vi "Graph_FPGA_v00.vi"() -> ()   [LabVIEW 2010]
doc: "Controls 6 phase locks based on the interference of two beams at a beam-splitter."
uses:
  Strict Type Defs/Graph Errors.ctl
  Strict Type Defs/Graph Lock Point.ctl
  Strict Type Defs/Graph Output.ctl
  Strict Type Defs/Control Graph Input.ctl
  Strict Type Defs/PII individual.ctl
  Strict Type Defs/Error Scale Graph.ctl
  Strict Type Defs/Lock Thresh Graph.ctl
  Strict Type Defs/Theta graph.ctl
  Strict Type Defs/Safety First.ctl
  Strict Type Defs/Scope.ctl
  Strict Type Defs/Graph Max.ctl
  Strict Type Defs/Graph Min.ctl
  <vilib>/eio/EIONode/EIONode.xnode
  <vilib>/rvi/eio/nirviEIOImplementation/nirviEIOImplementation.xnode
  <vilib>/rvi/eio/common/nirviEmuClasses.ctl
  <vilib>/rvi/DataTransferAndStorage/Container/XNode/niFpgaContainer.xnode
  <vilib>/rvi/DataTransferAndStorage/Container/Common/niFpgaContainerMethod.ctl
  <vilib>/rvi/DataTransferAndStorage/Container/Common/niFpgaTransferTypeControl.ctl
  <vilib>/rvi/eio/common/nirviEmuTemplateMethod_noerrors.vi
  <vilib>/rvi/interface/RandomDataEmulation/nirviRandomDataFPGAFIFO.vi
  <vilib>/rvi/interface/RandomDataEmulation/niFpgaRandomDataHandleErrors.vi
panel:
  out "PXI Trig 1":bool
  in  "Inverse":bool
  out "Measurement Tick Count(uSec)":u32
  in  "Measurement OFF (uSec)":u32 caption="Measurement OFF(uSec)"
  in  "offset time":u32
  out "Unlocked?(T=yes)":cluster{bool, bool, bool, bool, bool, bool}
  in  "RMS Thresh":T1={"Pump A"=2, "Pump B"=0, "EPR"=40, "Graph"=0, "HD A"=40, "HD B"=0}
  out "Min":T2
  out "Max":T3
  out "RMS Count":i32
  in  "RMS Stop":bool
  in  "Graph Delay(uSec)":u32 caption="Count(uSec)"
  out "HD Errors xp":T4
  in  "Scope":T5={"Trigger Direction"=enum."plus-minus", "Delay"=0, "Aquisition Rate (Ticks)"=40, "Offset"=0, "Channel"=0, "Channel Selector"={"Channel 1"=0, "Channel 2"=4, "Channel 3"=8, "Channel 4"=8}} {"Channel Selector"."Channel 4" items=["Error Signal 1", "Error Signal 2", "Scan Trigger 1", "Scan Trigger 2", "DC Signal 1", "DC Signal 2", "PI Out 1", "PI Out 2"]; "Channel Selector"."Channel 3" items=["Error Signal 1", "Error Signal 2", "Scan Trigger 1", "Scan Trigger 2", "DC Signal 1", "DC Signal 2", "PI Out 1", "PI Out 2"]; "Channel Selector"."Channel 2" items=["Error Signal 1", "Error Signal 2", "Scan Trigger 1", "Scan Trigger 2", "DC Signal 1", "DC Signal 2", "PI Out 1", "PI Out 2"]; "Channel Selector"."Channel 1" items=["Error Signal 1", "Error Signal 2", "Scan Trigger 1", "Scan Trigger 2", "DC Signal 1", "DC Signal 2", "PI Out 1", "PI Out 2"]}
  in  "quit Control Loop":bool
  in  "Control":T6={"PII In 1"={"Lock"=FALSE, "Hold"=FALSE, "P Gain"=0, "P BS"=-5, "I Gain"=0, "I BS"=-10, "I2 G"=0, "I2 BS"=-26, "Scan Amp"=0, "Scan Off"=0, "Scan FS"=0, "SFS BS"=0, "I Max value"=10000, "I2 Max value"=10000, "Scope.Offset"=0, "Trigger Direction"=enum."either", "Scan-PII thresh"=0}, "PII In 2"={"Lock"=FALSE, "Hold"=FALSE, "P Gain"=0, "P BS"=-10, "I Gain"=0, "I BS"=-10, "I2 G"=0, "I2 BS"=-26, "Scan Amp"=0, "Scan Off"=0, "Scan FS"=0, "SFS BS"=0, "I Max value"=10000, "I2 Max value"=10000, "Scope.Offset"=0, "Trigger Direction"=enum."either", "Scan-PII thresh"=0}, "PII In 3"={"Lock"=FALSE, "Hold"=FALSE, "P Gain"=0, "P BS"=-10, "I Gain"=0, "I BS"=-10, "I2 G"=0, "I2 BS"=-26, "Scan Amp"=0, "Scan Off"=0, "Scan FS"=0, "SFS BS"=0, "I Max value"=10000, "I2 Max value"=10000, "Scope.Offset"=0, "Trigger Direction"=enum."either", "Scan-PII thresh"=0}, "PII In 4"={"Lock"=FALSE, "Hold"=FALSE, "P Gain"=0, "P BS"=-10, "I Gain"=0, "I BS"=-10, "I2 G"=0, "I2 BS"=-26, "Scan Amp"=0, "Scan Off"=0, "Scan FS"=0, "SFS BS"=0, "I Max value"=10000, "I2 Max value"=10000, "Scope.Offset"=0, "Trigger Direction"=enum."either", "Scan-PII thresh"=0}, "PII In 5"={"Lock"=FALSE, "Hold"=FALSE, "P Gain"=10, "P BS"=-10, "I Gain"=0, "I BS"=0, "I2 G"=0, "I2 BS"=-26, "Scan Amp"=0, "Scan Off"=0, "Scan FS"=0, "SFS BS"=0, "I Max value"=10000, "I2 Max value"=10000, "Scope.Offset"=0, "Trigger Direction"=enum."either", "Scan-PII thresh"=0}, "PII In 6"={"Lock"=FALSE, "Hold"=FALSE, "P Gain"=0, "P BS"=-10, "I Gain"=0, "I BS"=-10, "I2 G"=0, "I2 BS"=-26, "Scan Amp"=0, "Scan Off"=0, "Scan FS"=0, "SFS BS"=0, "I Max value"=10000, "I2 Max value"=10000, "Scope.Offset"=0, "Trigger Direction"=enum."either", "Scan-PII thresh"=0}, "Error scale"={"Pre-Offset"={"Pre-Offset 1"=2, "Pre-Offset 2"=0, "Pre-Offset 3"=0, "Pre-Offset 4"=0, "Pre-Offset 5"=2, "Pre-Offset 6"=0, "Pre-Offset 7"=0, "Pre-Offset 8"=0}, "Post-Offset "={"Offset 1"=0, "Offset 2"=300, "Offset 3"=0, "Offset 4"=0, "Offset 5"=0, "Offset 6"=0, "Offset 7"=0, "Offset 8"=0}, "Gains"={"Gain 1"=0, "Gain 2"=300, "Gain 3"=0, "Gain 4"=0, "Gain 5"=0, "Gain 6"=0, "Gain 7"=0, "Gain 8"=0}, "Bit Shifts"={"Bit Shift 1"=0, "Bit Shift 2"=300, "Bit Shift 3"=0, "Bit Shift 4"=0, "Bit Shift 5"=0, "Bit Shift 6"=0, "Bit Shift 7"=0, "Bit Shift 8"=0}}, "Lock Thresh"={"Pump A"=0, "Pump B"=0, "EPR"=0, "Graph"=0, "HD A"=40, "HD B"=0}, "Re-Scan Thresh"={"Pump A"=2, "Pump B"=0, "EPR"=40, "Graph"=0, "HD A"=40, "HD B"=0}, "Theta"={"HD A Sin Theta"=0, "HD A Cos Theta"=0, "HD B Sin Theta"=0, "HD B Cos Theta"=0}, "Safety First"={"lim reset"=FALSE, "no limit"=FALSE, "pos slew rate * dt"=10, "neg slew rate * dt"=-10, "Hold All"=FALSE, "Count(Ticks)"=0}}
  in  "\"I too high?\"":T11
  in  "\"Outputs\"":T12
  out "Outputs":T12={"Pump A"=-270, "Pump B"=-1710, "EPR"=880, "Graph"=570, "HD A"=0, "HD B"=0}
  in  "\"Trigger\"":T11
  out "Trigger":T11
  out "Cavity Errors":T13={"Pump A"=0, "Pump B"=1800, "EPR"=0, "Graph"=0, "HD A"=0, "HD B"=0}
  out "Control Loop count":i32=11285327
  out "Scope Full?":bool
  out "Scope loop count":i32=119818
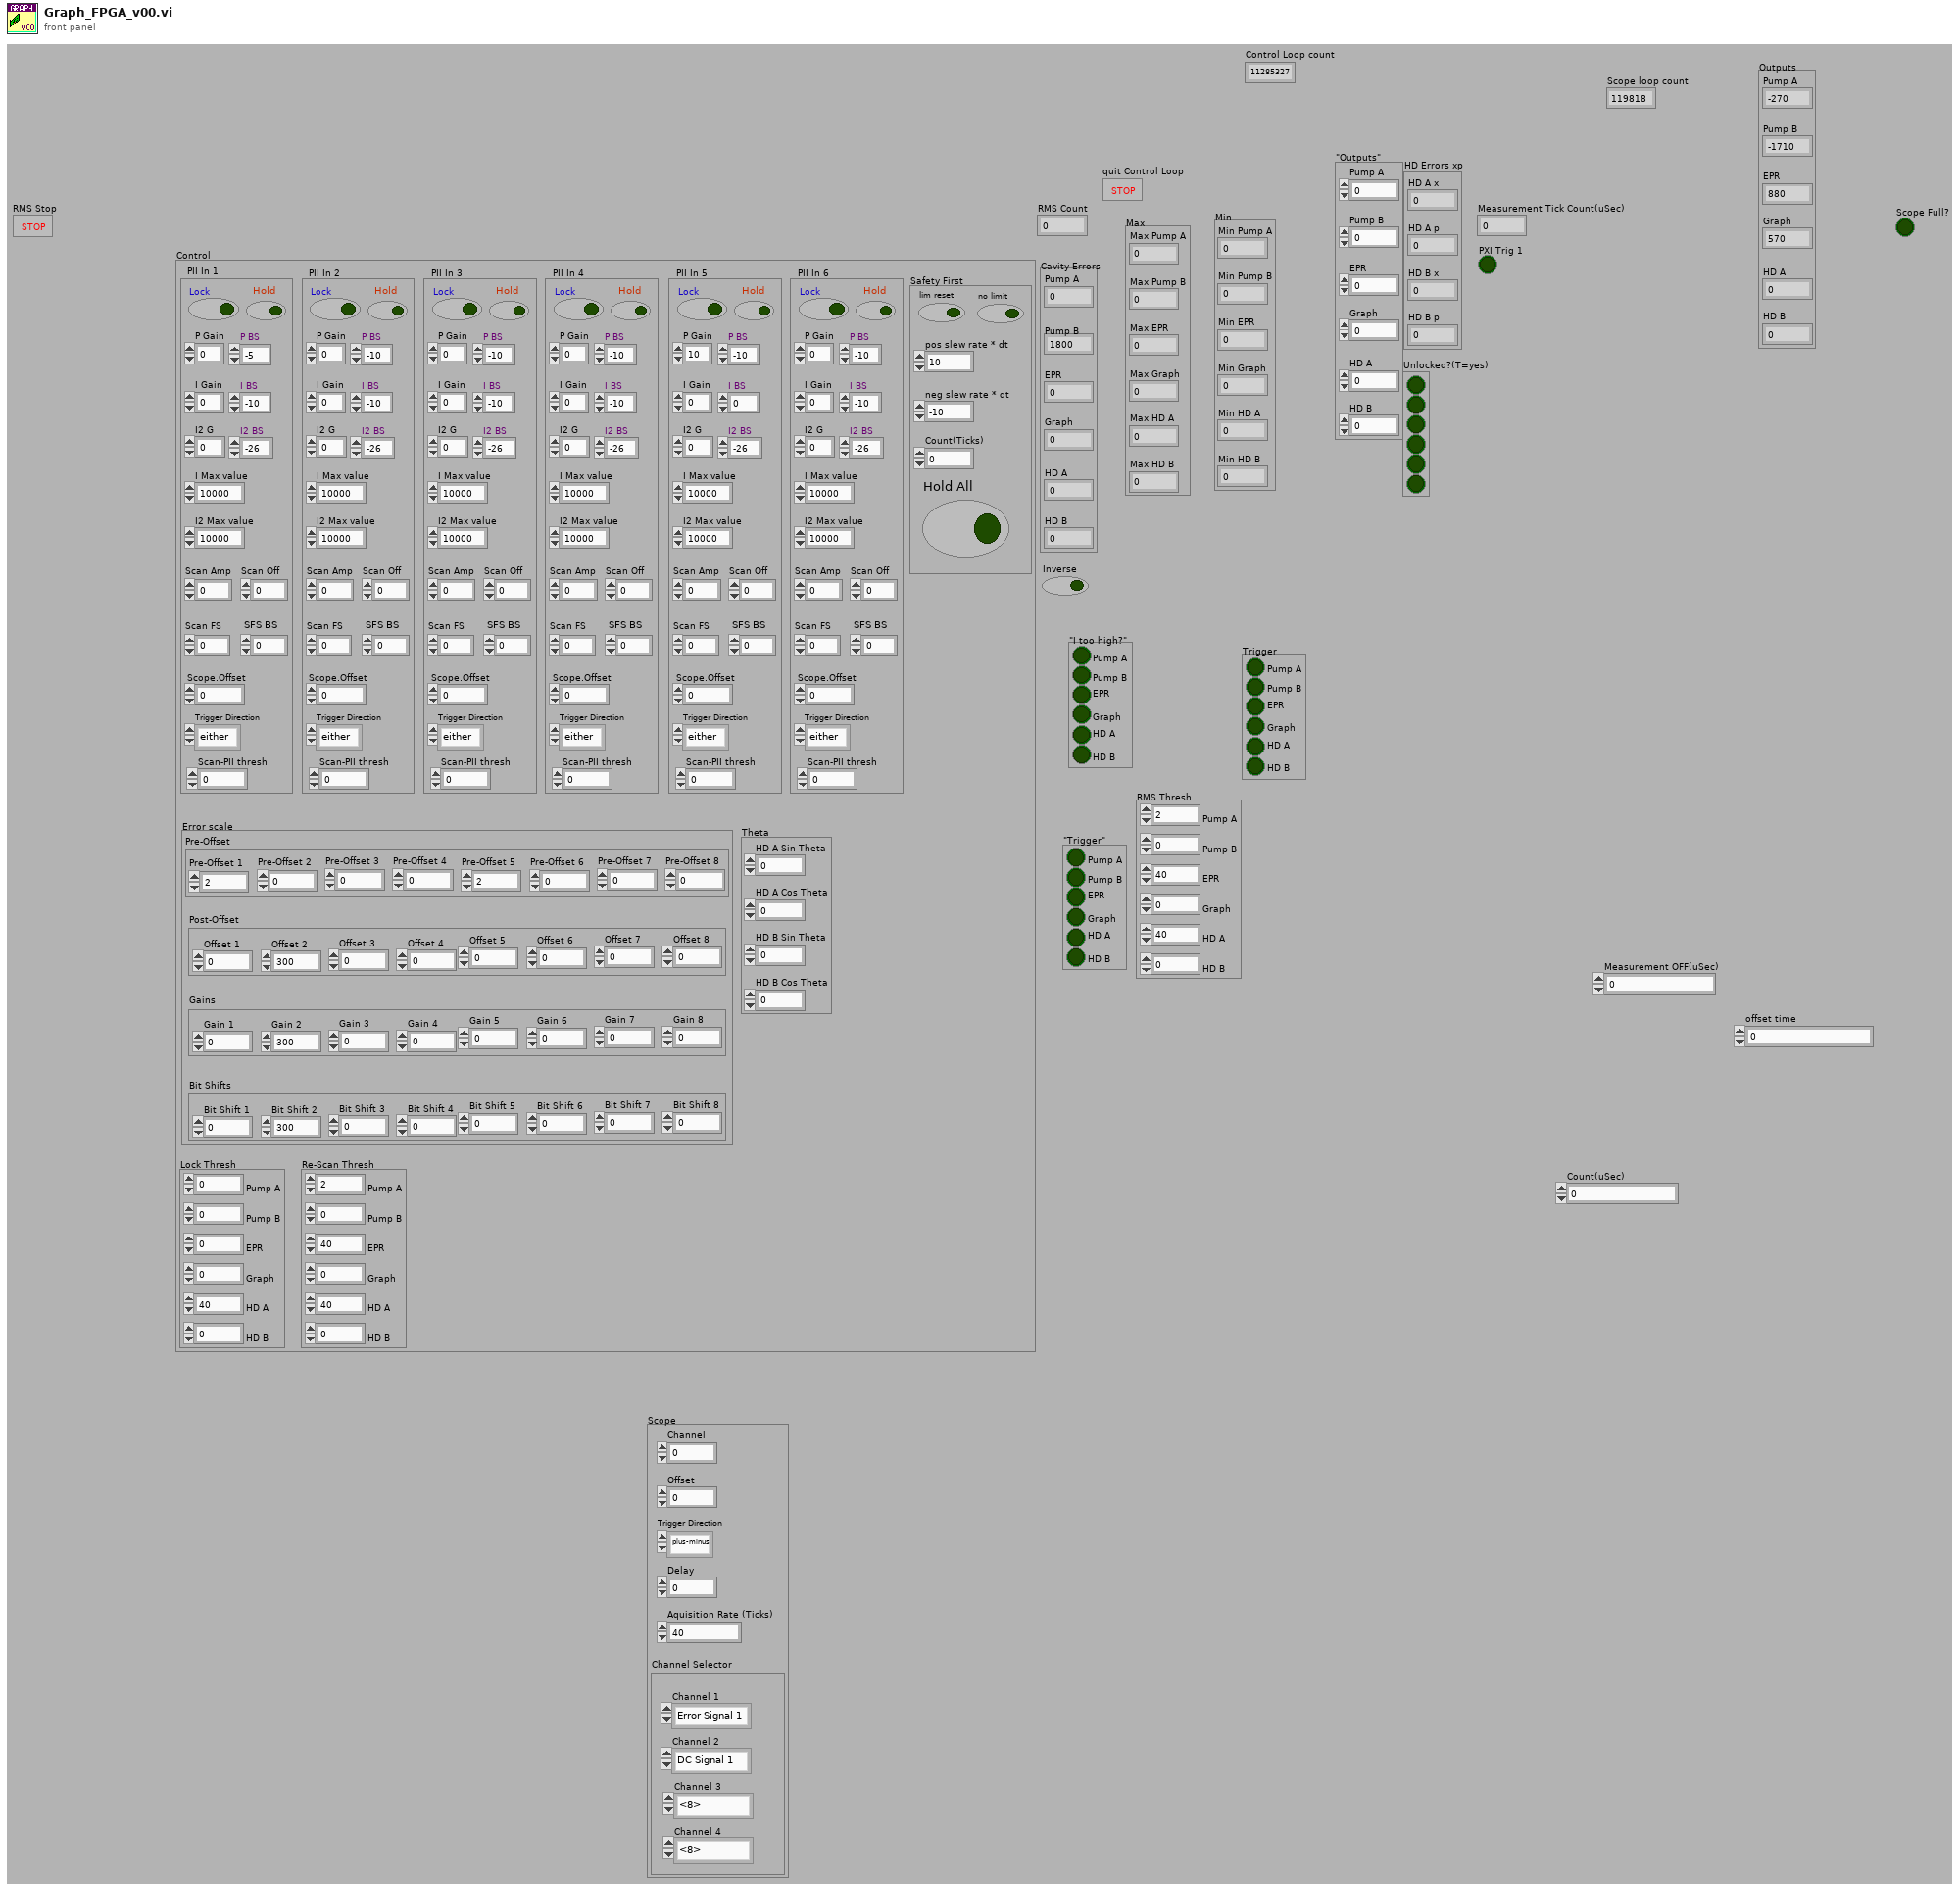
[diagram p1: front panel]
types:
  T1 = typedef "Lock Thresh Graph.ctl" = cluster{"Pump A":i16, "Pump B":i16, "EPR":i16, "Graph":i16, "HD A":i16, "HD B":i16}
  T2 = typedef "Graph Min.ctl" = cluster{"Min Pump A":i16, "Min Pump B":i16, "Min EPR":i16, "Min Graph":i16, "Min HD A":i16, "Min HD B":i16}
  T3 = typedef "Graph Max.ctl" = cluster{"Max Pump A":i16, "Max Pump B":i16, "Max EPR":i16, "Max Graph":i16, "Max HD A":i16, "Max HD B":i16}
  T4 = cluster{"HD A x":i16, "HD A p":i16, "HD B x":i16, "HD B p":i16}
  T5 = typedef "Scope.ctl" = cluster{"Trigger Direction":enum8{"either", "minus-plus", "plus-minus"}, "Delay":u32, "Aquisition Rate (Ticks)":u32, "Offset":i16, "Channel":i32, "Channel Selector":cluster{"Channel 1":i32, "Channel 2":i32, "Channel 3":i32, "Channel 4":i32}}
  T6 = typedef "Control Graph Input.ctl" = cluster{"PII In 1":T7, "PII In 2":T7, "PII In 3":T7, "PII In 4":T7, "PII In 5":T7, "PII In 6":T7, "Error scale":T8, "Lock Thresh":T1, "Re-Scan Thresh":T1, "Theta":T9, "Safety First":T10}
  T7 = typedef "PII individual.ctl" = cluster{"Lock":bool, "Hold":bool, "P Gain":i32, "P BS":i16, "I Gain":i32, "I BS":i16, "I2 G":i32, "I2 BS":i16, "Scan Amp":i16, "Scan Off":i16, "Scan FS":u16, "SFS BS":i16, "I Max value":i32, "I2 Max value":i32, "Scope.Offset":i16, "Trigger Direction":enum8{"either", "minus-plus", "plus-minus"}, "Scan-PII thresh":i16}
  T8 = typedef "Error Scale Graph.ctl" = cluster{"Pre-Offset":cluster{"Pre-Offset 1":i16, "Pre-Offset 2":i16, "Pre-Offset 3":i16, "Pre-Offset 4":i16, "Pre-Offset 5":i16, "Pre-Offset 6":i16, "Pre-Offset 7":i16, "Pre-Offset 8":i16}, "Post-Offset ":cluster{"Offset 1":i16, "Offset 2":i16, "Offset 3":i16, "Offset 4":i16, "Offset 5":i16, "Offset 6":i16, "Offset 7":i16, "Offset 8":i16}, "Gains":cluster{"Gain 1":i16, "Gain 2":i16, "Gain 3":i16, "Gain 4":i16, "Gain 5":i16, "Gain 6":i16, "Gain 7":i16, "Gain 8":i16}, "Bit Shifts":cluster{"Bit Shift 1":i16, "Bit Shift 2":i16, "Bit Shift 3":i16, "Bit Shift 4":i16, "Bit Shift 5":i16, "Bit Shift 6":i16, "Bit Shift 7":i16, "Bit Shift 8":i16}}
  T9 = typedef "Theta graph.ctl" = cluster{"HD A Sin Theta":i32, "HD A Cos Theta":i32, "HD B Sin Theta":i32, "HD B Cos Theta":i32}
  T10 = typedef "Safety First.ctl" = cluster{"lim reset":bool, "no limit":bool, "pos slew rate * dt":i16, "neg slew rate * dt":i16, "Hold All":bool, "Count(Ticks)":u32}
  T11 = typedef "Graph Lock Point.ctl" = cluster{"Pump A":bool, "Pump B":bool, "EPR":bool, "Graph":bool, "HD A":bool, "HD B":bool}
  T12 = typedef "Graph Output.ctl" = cluster{"Pump A":i16, "Pump B":i16, "EPR":i16, "Graph":i16, "HD A":i16, "HD B":i16}
  T13 = typedef "Graph Errors.ctl" = cluster{"Pump A":i16, "Pump B":i16, "EPR":i16, "Graph":i16, "HD A":i16, "HD B":i16}
  T14 = typedef "nirviEmuClasses.ctl" = enum16{"IO Read", "IO Write", "Method", "Property Read", "Property Write"}
  T15 = typedef "Signals Graph.ctl" = cluster{"PII In 1":T7, "PII In 2":T7, "PII In 3":T7, "PII In 4":T7, "PII In 5":T7, "PII In 6":T7, "Lock Thresh":T1, "Re-Scan Thresh":T1, "Safety First":T10, "Graph Errors":T13}
  T16 = typedef "Graph Control Cluster.ctl" = cluster{"Control Pump A":T7, "Control Pump B":T7, "Control EPR":T7, "Control Graph":T7, "Control HD A":T7, "Control HD B":T7, "Max":T3, "Min":T2, "Lock Threshold":T1, "Re-Scan Threshold":T1, "Lock Point?":T11, "Re-scan?":T11, "Lock pressed? (-1)":T11, "Cavity Errors":T13, "State (-1)":T17, "Safety First":T10}
  T17 = typedef "Graph State.ctl" = cluster{"Pump A":enum16{"Safe", "Hold", "Scan", "Lock"}, "Pump B":enum16{"Safe", "Hold", "Scan", "Lock"}, "EPR":enum16{"Safe", "Hold", "Scan", "Lock"}, "Graph":enum16{"Safe", "Hold", "Scan", "Lock"}, "HD A":enum16{"Safe", "Hold", "Scan", "Lock"}, "HD B":enum16{"Safe", "Hold", "Scan", "Lock"}}
  T18 = typedef "Graph PII Scan State.ctl" = cluster{"Control Pump A":T7, "Control Pump B":T7, "Control EPR":T7, "Control Graph":T7, "Control HD A":T7, "Control HD B":T7, "Error Signals":T13, "State":T17}
  T19 = typedef "Graph MaxMin.ctl" = cluster{"State":T17, "Reset MaxMin?":T20, "Max":T3, "Min":T2, "Lock pressed?":T11, "Safety First":T10}
  T20 = typedef "Graph Reset MaxMin.ctl" = cluster{"Pump A":bool, "Pump B":bool, "EPR":bool, "Graph":bool, "HD A":bool, "HD B":bool}
  T21 = typedef "niFpgaContainerMethod.ctl" = enum16{"<none>", "write", "read", "clear", "getNumberOfElementsToWrite", "getNumberOfElementsToRead", "enable", "disable", "flushAndDisable", "getStreamState", "readA", "readB", "dramWrite", "dramWriteWithByteEnables", "dramRequestData", "dramRetrieveData"}
  T22 = typedef "niFpgaTransferTypeControl.ctl" = enum16{"Target-Scoped", "Host to Target - DMA", "Target to Host - DMA", "Peer to Peer Reader", "Peer to Peer Writer", "Bidirectional"}
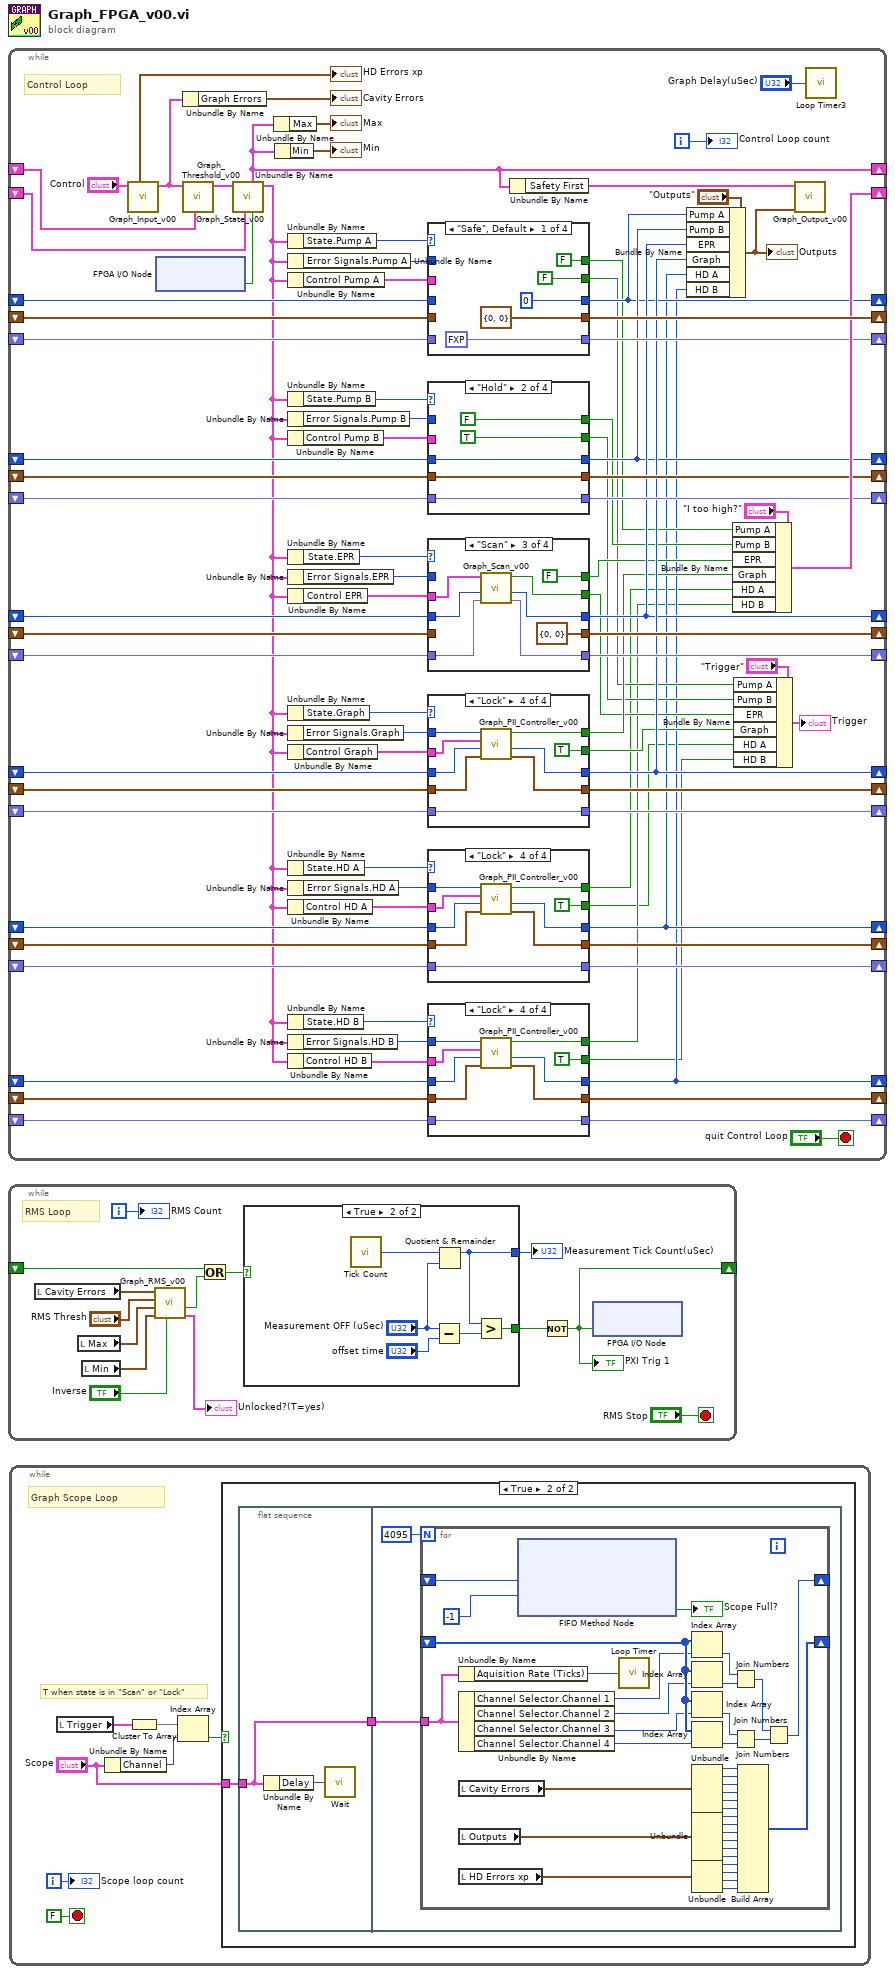
[diagram p0: block diagram]
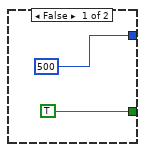
[diagram p2: hidden frame]
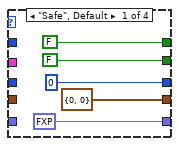
[diagram p4: hidden frame]
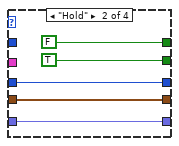
[diagram p5: hidden frame]
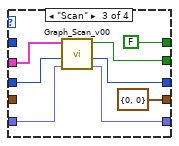
[diagram p6: hidden frame]
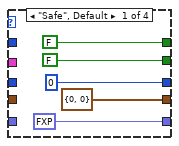
[diagram p7: hidden frame]
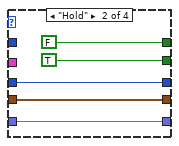
[diagram p8: hidden frame]
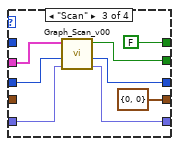
[diagram p9: hidden frame]
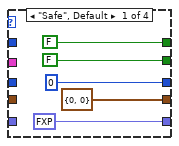
[diagram p10: hidden frame]
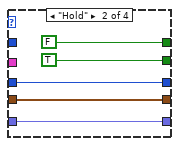
[diagram p11: hidden frame]
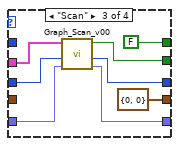
[diagram p12: hidden frame]
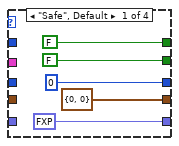
[diagram p13: hidden frame]
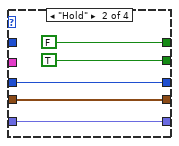
[diagram p14: hidden frame]
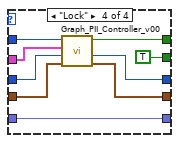
[diagram p15: hidden frame]
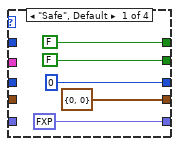
[diagram p16: hidden frame]
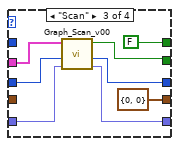
[diagram p17: hidden frame]
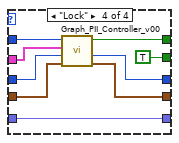
[diagram p18: hidden frame]
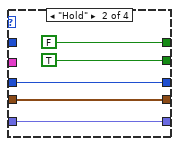
[diagram p19: hidden frame]
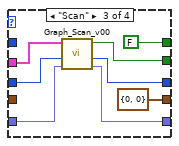
[diagram p20: hidden frame]
diagram:
  n1 = while {
    shift-right: [w87] -> _
    shift-left: _ -> [w85]
    shift-right: [w84] -> _
    shift-left: _ -> [w76]
    shift-right: [w54] -> _
    shift-left: _ -> [w86]
    shift-right: [w81] -> _
    shift-left: _ -> [w80]
    shift-right: [w21] -> _
    shift-left: _ -> [w75]
    shift-right: [w70] -> _
    shift-left: _ -> [w72]
    shift-right: [w55] -> _
    shift-left: _ -> [w71]
    shift-right: [w73] -> _
    shift-left: _ -> [w74]
    shift-right: [w69] -> _
    shift-left: _ -> [w67]
    shift-right: [w56] -> _
    shift-left: _ -> [w68]
    shift-right: [w66] -> _
    shift-left: _ -> [w65]
    shift-right: [w60] -> _
    shift-left: _ -> [w62]
    shift-right: [w57] -> _
    shift-left: _ -> [w61]
    shift-right: [w63] -> _
    shift-left: _ -> [w64]
    shift-right: [w43] -> _
    shift-left: _ -> [w41]
    shift-right: [w33] -> _
    shift-left: _ -> [w42]
    shift-right: [w40] -> _
    shift-left: _ -> [w39]
    shift-right: [w34] -> _
    shift-left: _ -> [w36]
    shift-right: [w32] -> _
    shift-left: _ -> [w35]
    shift-right: [w37] -> _
    shift-left: _ -> [w38]
    i -> [w77]
    stop <- "quit Control Loop" stop-if-true
    # "Control Loop"
    n2 = call "Graph_Input_v00.vi"("Control"="Control") -> ("Signals"=w27:T15, "HD Errors xp"=→"HD Errors xp":T4)  [unwired: 9 in]
    n3 = xnode "FPGA I/O Node"() -> ("PXI_Trig0"=w24:bool)  [unwired: 1 in, 1 out]
    n4 = Unbundle By Name(w27) -> ("Graph Errors"=→"Cavity Errors":T13)
    n5 = call "Graph_Threshold_v00.vi"("MaxMin"=w75, "Signals"=w27) -> ("Control Graph Cluster"=w23:T16)  [unwired: 9 in]
    n6 = call "Graph_State_v00.vi"("BS Hold Pulse"=w24, "\"I too high?\""=w76, "Control Cavity Cluster"=w23) -> ("PII Scan State Errors"=w1:T18, "MaxMin"=w21:T19)  [unwired: 7 in]
    n7 = Unbundle By Name(w21) -> ("Max"=→"Max":T3)
    n8 = Unbundle By Name(w21) -> ("Min"=→"Min":T2)
    n9 = Unbundle By Name(w1) -> ("State.Pump A"=w18:enum16{"Safe", "Hold", "Scan", "Lock"})
    n10 = Unbundle By Name(w1) -> ("Error Signals.Pump A"=w19:i16)
    n11 = Unbundle By Name(w1) -> ("Control Pump A"=w17:T7)
    n12 = Unbundle By Name(w1) -> ("State.Pump B"=w15:enum16{"Safe", "Hold", "Scan", "Lock"})
    n13 = Unbundle By Name(w1) -> ("Error Signals.Pump B"=w16:i16)
    n14 = Unbundle By Name(w1) -> ("Control Pump B"=w14:T7)
    n15 = Unbundle By Name(w1) -> ("State.EPR"=w11:enum16{"Safe", "Hold", "Scan", "Lock"})
    n16 = Unbundle By Name(w1) -> ("Error Signals.EPR"=w12:i16)
    n17 = Unbundle By Name(w1) -> ("Control EPR"=w13:T7)
    n18 = Unbundle By Name(w1) -> ("State.Graph"=w9:enum16{"Safe", "Hold", "Scan", "Lock"})
    n19 = Unbundle By Name(w1) -> ("Error Signals.Graph"=w10:i16)
    n20 = Unbundle By Name(w1) -> ("Control Graph"=w8:T7)
    n21 = Unbundle By Name(w1) -> ("State.HD A"=w7:enum16{"Safe", "Hold", "Scan", "Lock"})
    n22 = Unbundle By Name(w1) -> ("Error Signals.HD A"=w6:i16)
    n23 = Unbundle By Name(w1) -> ("Control HD A"=w5:T7)
    n24 = Unbundle By Name(w1) -> ("State.HD B"=w2:enum16{"Safe", "Hold", "Scan", "Lock"})
    n25 = Unbundle By Name(w1) -> ("Error Signals.HD B"=w4:i16)
    n26 = Unbundle By Name(w1) -> ("Control HD B"=w3:T7)
    n27 = case shown="\"Safe\", Default" w18 {
      tunnel: w19 -> [_ _ _ w269]
      tunnel: [cluster{"I Cavity":i32, "I2 Cavity":i32} {"I Cavity"=0, "I2 Cavity"=0} ("Integrator") w250 cluster{"I Cavity":i32, "I2 Cavity":i32} {"I Cavity"=0, "I2 Cavity"=0} ("Integrator") w265] -> w87
      tunnel: [FALSE ("I too high? (F=No)") FALSE ("I too high? (F=No)") FALSE ("I too high? (F=No)") w268] -> w53
      tunnel: w17 -> [_ _ w259 w266]
      tunnel: [i16 0 ("PII out") w251 w258 w262] -> w54
      tunnel: w86 -> [_ w251 w255 w263]
      tunnel: w85 -> [_ w250 _ w267]
      tunnel: [fxp<+,33,17> 0.0 ("Scan") w249 w257 w261] -> w81
      tunnel: w80 -> [_ w249 w256 w261]
      tunnel: [FALSE ("Zero Crossing") TRUE ("Zero Crossing") w254 TRUE ("Zero Crossing")] -> w49
      frame "Safe", Default {
      }
      frame "Hold" {
      }
      frame "Scan" {
        n28 = call "Graph_Scan_v00.vi"("Scan (-1)"=w256, "Scan out (-1)"=w255, "Control Cavity"=w259) -> ("Scan"=w257:fxp<+,33,17>, "Scan out"=w258:i16, "Zero Crossing"=w254:bool)  [unwired: 6 in]
      }
      frame "Lock" {
        n29 = call "Graph_PII_Controller_v00.vi"("Integrator (-1)"=w267, "PII out (-1)"=w263, "Control Cavity"=w266, "OPO A Error"=w269) -> ("Integrator"=w265:cluster{"I Cavity":i32, "I2 Cavity":i32}, "PII out"=w262:i16, "I too high?"=w268:bool)  [unwired: 5 in]
      }
    }
    n30 = case shown="\"Hold\"" w15 {
      tunnel: w16 -> [_ _ _ w242]
      tunnel: [cluster{"I Cavity":i32, "I2 Cavity":i32} {"I Cavity"=0, "I2 Cavity"=0} ("Integrator") w223 cluster{"I Cavity":i32, "I2 Cavity":i32} {"I Cavity"=0, "I2 Cavity"=0} ("Integrator") w238] -> w70
      tunnel: [FALSE ("I too high? (F=No)") FALSE ("I too high? (F=No)") FALSE ("I too high? (F=No)") w241] -> w52
      tunnel: w14 -> [_ _ w232 w239]
      tunnel: [i16 0 ("PII out") w224 w231 w236] -> w55
      tunnel: w71 -> [_ w224 w228 w237]
      tunnel: w72 -> [_ w223 _ w240]
      tunnel: [fxp<+,33,17> 0.0 ("Scan") w222 w230 w235] -> w73
      tunnel: w74 -> [_ w222 w229 w235]
      tunnel: [FALSE ("Zero Crossing") TRUE ("Zero Crossing") w226 TRUE ("Zero Crossing")] -> w45
      frame "Safe", Default {
      }
      frame "Hold" {
      }
      frame "Scan" {
        n31 = call "Graph_Scan_v00.vi"("Scan (-1)"=w229, "Scan out (-1)"=w228, "Control Cavity"=w232) -> ("Scan"=w230:fxp<+,33,17>, "Scan out"=w231:i16, "Zero Crossing"=w226:bool)  [unwired: 6 in]
      }
      frame "Lock" {
        n32 = call "Graph_PII_Controller_v00.vi"("Integrator (-1)"=w240, "PII out (-1)"=w237, "Control Cavity"=w239, "OPO A Error"=w242) -> ("Integrator"=w238:cluster{"I Cavity":i32, "I2 Cavity":i32}, "PII out"=w236:i16, "I too high?"=w241:bool)  [unwired: 5 in]
      }
    }
    n33 = case shown="\"Scan\"" w11 {
      tunnel: w12 -> [_ _ _ w215]
      tunnel: [cluster{"I Cavity":i32, "I2 Cavity":i32} {"I Cavity"=0, "I2 Cavity"=0} ("Integrator") w196 cluster{"I Cavity":i32, "I2 Cavity":i32} {"I Cavity"=0, "I2 Cavity"=0} ("Integrator") w211] -> w69
      tunnel: [FALSE ("I too high? (F=No)") FALSE ("I too high? (F=No)") FALSE ("I too high? (F=No)") w214] -> w51
      tunnel: w13 -> [_ _ w205 w212]
      tunnel: [i16 0 ("PII out") w197 w204 w208] -> w56
      tunnel: w68 -> [_ w197 w201 w209]
      tunnel: w67 -> [_ w196 _ w213]
      tunnel: [fxp<+,33,17> 0.0 ("Scan") w195 w203 w207] -> w66
      tunnel: w65 -> [_ w195 w202 w207]
      tunnel: [FALSE ("Zero Crossing") TRUE ("Zero Crossing") w200 TRUE ("Zero Crossing")] -> w48
      frame "Safe", Default {
      }
      frame "Hold" {
      }
      frame "Scan" {
        n34 = call "Graph_Scan_v00.vi"("Scan (-1)"=w202, "Scan out (-1)"=w201, "Control Cavity"=w205) -> ("Scan"=w203:fxp<+,33,17>, "Scan out"=w204:i16, "Zero Crossing"=w200:bool)  [unwired: 6 in]
      }
      frame "Lock" {
        n35 = call "Graph_PII_Controller_v00.vi"("Integrator (-1)"=w213, "PII out (-1)"=w209, "Control Cavity"=w212, "OPO A Error"=w215) -> ("Integrator"=w211:cluster{"I Cavity":i32, "I2 Cavity":i32}, "PII out"=w208:i16, "I too high?"=w214:bool)  [unwired: 5 in]
      }
    }
    n36 = case shown="\"Lock\"" w9 {
      tunnel: w10 -> [_ _ _ w188]
      tunnel: [cluster{"I Cavity":i32, "I2 Cavity":i32} {"I Cavity"=0, "I2 Cavity"=0} ("Integrator") w169 cluster{"I Cavity":i32, "I2 Cavity":i32} {"I Cavity"=0, "I2 Cavity"=0} ("Integrator") w184] -> w60
      tunnel: [FALSE ("I too high? (F=No)") FALSE ("I too high? (F=No)") FALSE ("I too high? (F=No)") w187] -> w50
      tunnel: w8 -> [_ _ w178 w185]
      tunnel: [i16 0 ("PII out") w170 w177 w181] -> w57
      tunnel: w61 -> [_ w170 w174 w182]
      tunnel: w62 -> [_ w169 _ w186]
      tunnel: [fxp<+,33,17> 0.0 ("Scan") w168 w176 w180] -> w63
      tunnel: w64 -> [_ w168 w175 w180]
      tunnel: [FALSE ("Zero Crossing") TRUE ("Zero Crossing") w173 TRUE ("Zero Crossing")] -> w47
      frame "Safe", Default {
      }
      frame "Hold" {
      }
      frame "Scan" {
        n37 = call "Graph_Scan_v00.vi"("Scan (-1)"=w175, "Scan out (-1)"=w174, "Control Cavity"=w178) -> ("Scan"=w176:fxp<+,33,17>, "Scan out"=w177:i16, "Zero Crossing"=w173:bool)  [unwired: 6 in]
      }
      frame "Lock" {
        n38 = call "Graph_PII_Controller_v00.vi"("Integrator (-1)"=w186, "PII out (-1)"=w182, "Control Cavity"=w185, "OPO A Error"=w188) -> ("Integrator"=w184:cluster{"I Cavity":i32, "I2 Cavity":i32}, "PII out"=w181:i16, "I too high?"=w187:bool)  [unwired: 5 in]
      }
    }
    n39 = case shown="\"Lock\"" w7 {
      tunnel: w6 -> [_ _ _ w161]
      tunnel: [cluster{"I Cavity":i32, "I2 Cavity":i32} {"I Cavity"=0, "I2 Cavity"=0} ("Integrator") w142 cluster{"I Cavity":i32, "I2 Cavity":i32} {"I Cavity"=0, "I2 Cavity"=0} ("Integrator") w157] -> w43
      tunnel: [FALSE ("I too high? (F=No)") FALSE ("I too high? (F=No)") FALSE ("I too high? (F=No)") w160] -> w31
      tunnel: w5 -> [_ _ w151 w158]
      tunnel: [i16 0 ("PII out") w143 w150 w154] -> w33
      tunnel: w42 -> [_ w143 w147 w155]
      tunnel: w41 -> [_ w142 _ w159]
      tunnel: [fxp<+,33,17> 0.0 ("Scan") w141 w149 w153] -> w40
      tunnel: w39 -> [_ w141 w148 w153]
      tunnel: [FALSE ("Zero Crossing") TRUE ("Zero Crossing") w146 TRUE ("Zero Crossing")] -> w29
      frame "Safe", Default {
      }
      frame "Hold" {
      }
      frame "Scan" {
        n40 = call "Graph_Scan_v00.vi"("Scan (-1)"=w148, "Scan out (-1)"=w147, "Control Cavity"=w151) -> ("Scan"=w149:fxp<+,33,17>, "Scan out"=w150:i16, "Zero Crossing"=w146:bool)  [unwired: 6 in]
      }
      frame "Lock" {
        n41 = call "Graph_PII_Controller_v00.vi"("Integrator (-1)"=w159, "PII out (-1)"=w155, "Control Cavity"=w158, "OPO A Error"=w161) -> ("Integrator"=w157:cluster{"I Cavity":i32, "I2 Cavity":i32}, "PII out"=w154:i16, "I too high?"=w160:bool)  [unwired: 5 in]
      }
    }
    n42 = case shown="\"Lock\"" w2 {
      tunnel: w4 -> [_ _ _ w134]
      tunnel: [cluster{"I Cavity":i32, "I2 Cavity":i32} {"I Cavity"=0, "I2 Cavity"=0} ("Integrator") w115 cluster{"I Cavity":i32, "I2 Cavity":i32} {"I Cavity"=0, "I2 Cavity"=0} ("Integrator") w130] -> w34
      tunnel: [FALSE ("I too high? (F=No)") FALSE ("I too high? (F=No)") FALSE ("I too high? (F=No)") w133] -> w30
      tunnel: w3 -> [_ _ w124 w131]
      tunnel: [i16 0 ("PII out") w116 w123 w127] -> w32
      tunnel: w35 -> [_ w116 w120 w128]
      tunnel: w36 -> [_ w115 _ w132]
      tunnel: [fxp<+,33,17> 0.0 ("Scan") w114 w122 w126] -> w37
      tunnel: w38 -> [_ w114 w121 w126]
      tunnel: [FALSE ("Zero Crossing") TRUE ("Zero Crossing") w119 TRUE ("Zero Crossing")] -> w28
      frame "Safe", Default {
      }
      frame "Hold" {
      }
      frame "Scan" {
        n43 = call "Graph_Scan_v00.vi"("Scan (-1)"=w121, "Scan out (-1)"=w120, "Control Cavity"=w124) -> ("Scan"=w122:fxp<+,33,17>, "Scan out"=w123:i16, "Zero Crossing"=w119:bool)  [unwired: 6 in]
      }
      frame "Lock" {
        n44 = call "Graph_PII_Controller_v00.vi"("Integrator (-1)"=w132, "PII out (-1)"=w128, "Control Cavity"=w131, "OPO A Error"=w134) -> ("Integrator"=w130:cluster{"I Cavity":i32, "I2 Cavity":i32}, "PII out"=w127:i16, "I too high?"=w133:bool)  [unwired: 5 in]
      }
    }
    n45 = Unbundle By Name(w21) -> ("Safety First"=w59:T10)
    n46 = Bundle By Name(cluster="\"Outputs\"", "Pump A"=w54, "Pump B"=w55, "EPR"=w56, "Graph"=w57, "HD A"=w33, "HD B"=w32) -> (w58:T12)
    "Outputs" <- w58
    n47 = Bundle By Name(cluster="\"I too high?\"", "Pump A"=w53, "Pump B"=w52, "EPR"=w51, "Graph"=w50, "HD A"=w31, "HD B"=w30) -> (w84:T11)
    n48 = Bundle By Name(cluster="\"Trigger\"", "Pump A"=w49, "Pump B"=w45, "EPR"=w48, "Graph"=w47, "HD A"=w29, "HD B"=w28) -> (→"Trigger":T11)
    n49 = call "Graph_Output_v00.vi"("Outputs"=w58, "Safety First"=w59) -> ()  [unwired: 10 in]
    n50 = call "Loop Timer3"("Count(uSec)"="Graph Delay(uSec)") -> ()  [unwired: 1 out]
    "Control Loop count" <- w77
  }
  n51 = while {
    shift-right: [w271] -> _
    shift-left: _ -> [w273]
    i -> [w282]
    stop <- "RMS Stop" stop-if-true
    # "RMS Loop"
    n52 = local read "Cavity Errors"() -> (w281:T13)
    n53 = local read "Max"() -> (w279:T3)
    n54 = local read "Min"() -> (w278:T2)
    n55 = call "Graph_RMS_v00.vi"("Inverse"="Inverse", "Min"=w278, "Max"=w279, "RMS Thresh"="RMS Thresh", "Cavity Errors"=w281) -> ("UnlLocked?(T=yes)"=→"Unlocked?(T=yes)":cluster{bool, bool, bool, bool, bool, bool}, "Unlocked?(T=Don`t measure)"=w275:bool)  [unwired: 5 in]
    n56 = Or(x=w273, y=w275) -> (x .or. y?=w276:bool)
    n57 = case shown="True" w276 {
      tunnel: [TRUE ("t") w286] -> w274
      tunnel: [u32 500 ("Tick Count(uSec)") w290] -> w272
      frame False {
      }
      frame True {
        n58 = call "Tick Count"() -> ("Tick Count(uSec)"=w291:u32)
        n59 = Subtract(x="Measurement OFF (uSec)", y="offset time") -> (x-y=w287:u32)
        n60 = Quotient & Remainder(x=w291, y="Measurement OFF (uSec)") -> (x-y*floor(x/y)=w290:u32)  [unwired: 1 out]
        n61 = Greater?(x=w290, y=w287) -> (0:w286:bool)
      }
    }
    "Measurement Tick Count(uSec)" <- w272
    n62 = Not(x=w274) -> (.not. x?=w271:bool)
    "PXI Trig 1" <- w271
    n63 = xnode "FPGA I/O Node"("PXI_Trig1"=w271) -> ()  [unwired: 1 in, 1 out]
    "RMS Count" <- w282
  }
  n64 = while {
    i -> [w306]
    stop <- FALSE ("stop") stop-if-true
    # "Graph Scope Loop"
    # "T when state is in \"Scan\" or \"Lock\""
    n65 = local read "Trigger"() -> (w304:T11)
    n66 = Unbundle By Name("Scope") -> ("Channel"=w307:i32)
    n67 = Cluster To Array(cluster=w304) -> (array=w308:bool[])
    n68 = Index Array(array=w308, index=w307) -> (element=w305:bool)
    n69 = case shown="True" w305 {
      tunnel: "Scope" -> [_ w311]
      frame False {
      }
      frame True {
        n70 = flat-sequence {
          tunnel: w311 -> [w312]
          tunnel: [w312] -> w310
          tunnel: w310 -> [w314]
          frame #0 {
            n71 = Unbundle By Name(w312) -> ("Delay"=w313:u32)
            n72 = call "Wait"("Count(Ticks)"=w313) -> ()  [unwired: 1 out]
          }
          frame #1 {
            n73 = for {
              N: 4095 -> [_]
              tunnel: w314 -> [w351]
              shift-right: [w343] -> _
              shift-left: _ -> [w342]
              shift-right: [w338] -> _
              shift-left: _ -> [w337]
              n74 = Unbundle By Name(w351) -> ("Aquisition Rate (Ticks)"=w352:u32)
              n75 = Unbundle By Name(w351) -> ("Channel Selector.Channel 1"=w339:i32, "Channel Selector.Channel 2"=w340:i32, "Channel Selector.Channel 3"=w334:i32, "Channel Selector.Channel 4"=w341:i32)
              n76 = local read "Cavity Errors"() -> (w350:T13)
              n77 = local read "Outputs"() -> (w349:T12)
              n78 = local read "HD Errors xp"() -> (w332:T4)
              n79 = xnode ("FIFO Method Node")("Element"=w337, "Timeout"=-1) -> ("Timed Out?"=→"Scope Full?":bool)  [unwired: 1 in, 1 out]
              n80 = call "Loop Timer"("Count(uSec)"=w352) -> ()  [unwired: 1 out]
              n81 = Index Array(array=w342, index=w339) -> (element=w345:i16)
              n82 = Index Array(array=w342, index=w340) -> (element=w344:i16)
              n83 = Index Array(array=w342, index=w334) -> (element=w333:i16)
              n84 = Index Array(array=w342, index=w341) -> (element=w346:i16)
              n85 = Unbundle(w350) -> ("Pump A"=w331:i16, "Pump B"=w330:i16, "EPR"=w329:i16, "Graph"=w328:i16, "HD A"=w327:i16, "HD B"=w326:i16)
              n86 = Unbundle(w349) -> ("Pump A"=w325:i16, "Pump B"=w324:i16, "EPR"=w323:i16, "Graph"=w322:i16, "HD A"=w321:i16, "HD B"=w320:i16)
              n87 = Unbundle(w332) -> ("HD A x"=w319:i16, "HD A p"=w318:i16, "HD B x"=w317:i16, "HD B p"=w316:i16)
              n88 = Join Numbers(hi=w345, lo=w344) -> ((hi.lo)=w348:u32)
              n89 = Join Numbers(hi=w333, lo=w346) -> ((hi.lo)=w347:u32)
              n90 = Build Array(w331, w330, w329, w328, w327, w326, w325, w324, w323, w322, w321, w320, w319, w318, w317, w316) -> (w343:i16[])
              n91 = Join Numbers(hi=w348, lo=w347) -> ((hi.lo)=w338:u64)
            }
          }
        }
      }
    }
    "Scope loop count" <- w306
  }
